vi "定点周期设置.vi"(10 "配置信息":T9, 11 "测试状态输入":T1) -> (2 "周期设置输出":T10, 3 "测试状态输出":T1)   [LabVIEW 2016, in "TimingControl.lvclass"]
uses:
  TimingControl.lvclass
  <vilib>/Utility/miscctls.llb/LVPointTypeDef.ctl
panel:
  in  "每月启动":T3
  in  "每周启动":T2
  out "测试状态.结束时间":timestamp caption="结束时间" format="%<%y/%m/%d %H:%M:%S>T"
  out "测试状态.启动次数":dbl caption="启动次数"
  out "测试状态.启动时间":timestamp caption="启动时间" format="%<%y/%m/%d %H:%M:%S>T"
  in  "测量参数":T5 items=["氨氮"]
  out "保存输出":bool
  in  "保存":bool
  in  "退出":bool
  in  "批量设置":bool
  out "周期模式选择卡":enum32{"选项卡 1", "选项卡 2"}(tab)
  in  "定点周期":T6
  in  "间隔启动":T8
  in  "周期模式":T4
  # "分钟"
  # "次"
  # "分钟"
  # "次"
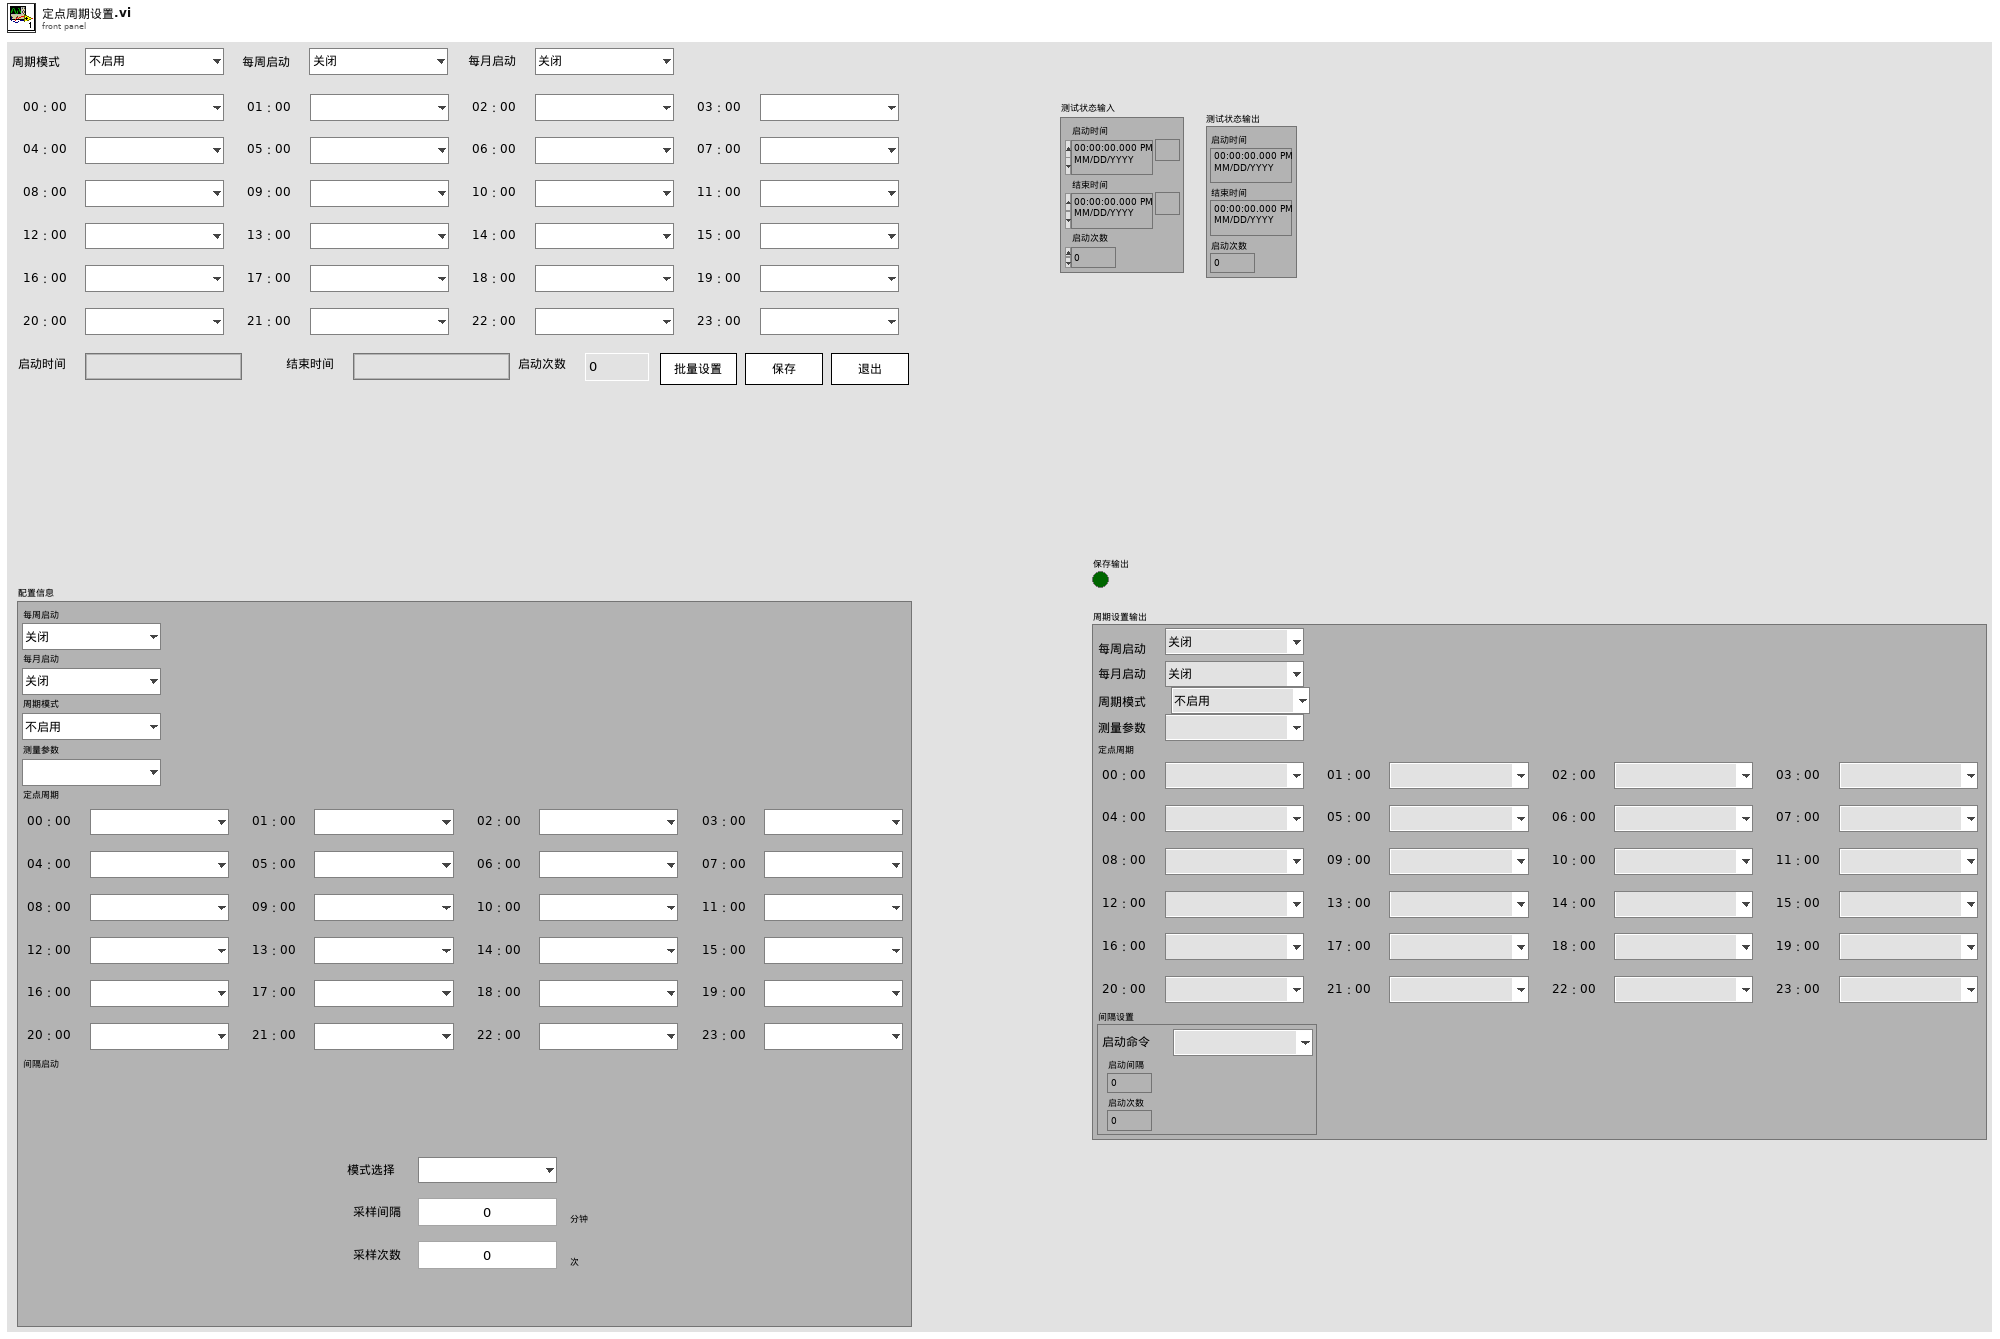
[diagram p1: front panel]
types:
  T1 = cluster{"启动时间":timestamp, "结束时间":timestamp, "启动次数":dbl}
  T2 = typedef "TimingControl.lvclass/每周启动.ctl" = enum16{"关闭", "周日", "周一", "周二", "周三", "周四", "周五", "周六"}
  T3 = typedef "TimingControl.lvclass/每月启动.ctl" = enum16{"关闭", "1号", "2号", "3号", "4号", "5号", "6号", "7号", "8号", "9号", "10号", "11号", "12号", "13号", "14号", "15号", "16号", "17号", "18号", "19号", "20号", "21号", "22号", "23号", "24号", "25号", "26号", "27号", "28号", "29号", "30号", "31号"}
  T4 = typedef "TimingControl.lvclass/周期模式设置.ctl" = enum16{"不启用", "定点模式", "间隔模式"}
  T5 = typedef "TimingControl.lvclass/测量参数.ctl" = u16
  T6 = typedef "TimingControl.lvclass/定点周期设置.ctl" = cluster{"启动命令":T7, "启动命令 2":T7, "启动命令 3":T7, "启动命令 4":T7, "启动命令 5":T7, "启动命令 6":T7, "启动命令 7":T7, "启动命令 8":T7, "启动命令 9":T7, "启动命令 10":T7, "启动命令 11":T7, "启动命令 12":T7, "启动命令 13":T7, "启动命令 14":T7, "启动命令 15":T7, "启动命令 16":T7, "启动命令 17":T7, "启动命令 18":T7, "启动命令 19":T7, "启动命令 20":T7, "启动命令 21":T7, "启动命令 22":T7, "启动命令 23":T7, "启动命令 24":T7}
  T7 = typedef "TimingControl.lvclass/启动命令选择.ctl" = enum16{"", "水样测试", "标样核查", "零点核查", "跨度核查", "空白测试", "平行样测试", "加标回收", "空白校准", "标样校准", "初始化(清洗)"}
  T8 = typedef "TimingControl.lvclass/间隔启动设置.ctl" = cluster{"启动命令":T7, "启动间隔":dbl, "启动次数":i32}
  T9 = cluster{"每周启动":T2, "每月启动":T3, "周期模式":T4, "测量参数":T5, "定点周期":T6, "间隔启动":T8}
  T10 = cluster{"每周启动":T2, "每月启动":T3, "周期模式":T4, "测量参数":T5, "定点周期":T6, "间隔设置":cluster{"启动命令":T7, "启动间隔":dbl, "启动次数":i32}}
  T11 = typedef "LVPointTypeDef.ctl" = cluster{"Horizontal":i16, "Vertical":i16}
  T12 = typedef "周期设置.lvlib/周期模式设置.ctl" = enum16{"不启用", "定点模式", "间隔模式"}
  T13 = cluster{"每周启动":T2, "每月启动":T3, "周期模式":T4, "测量参数":T5, "定点周期":T6, cluster{"启动命令":T7, "启动间隔":dbl, "启动次数":i32}}
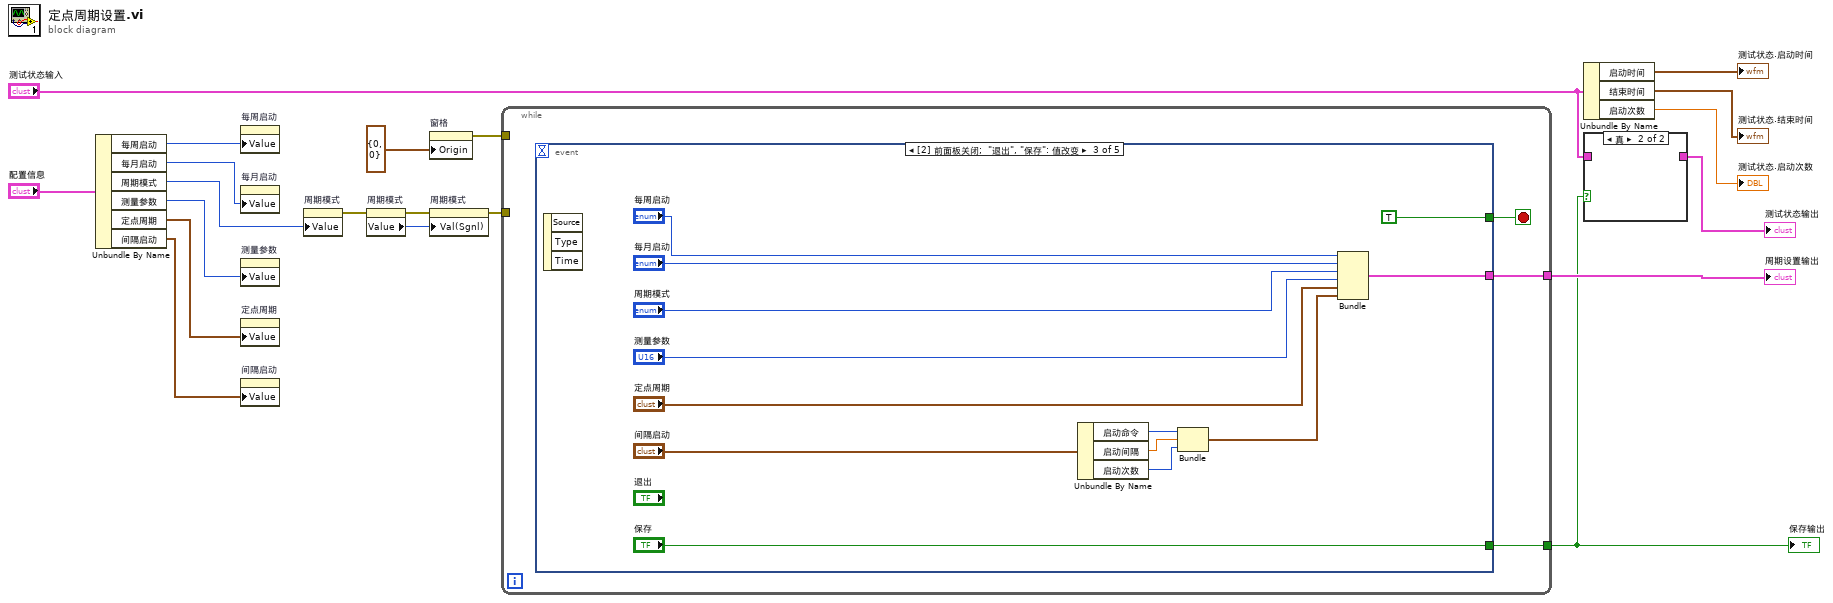
[diagram p0: block diagram]
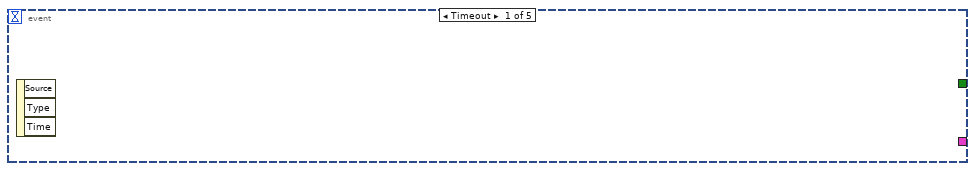
[diagram p3: hidden frame]
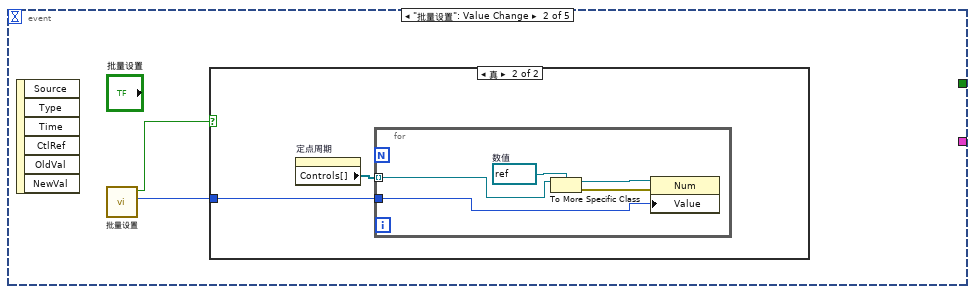
[diagram p4: hidden frame]
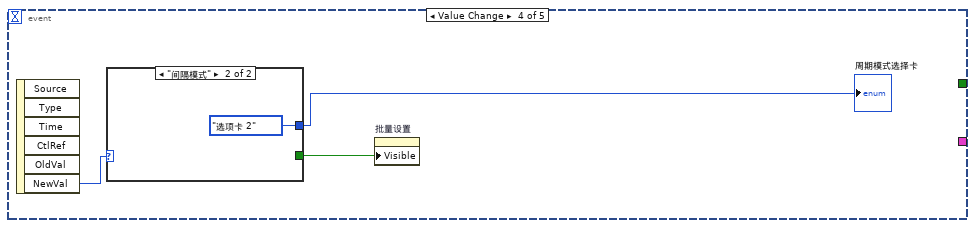
[diagram p6: hidden frame]
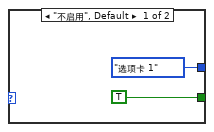
[diagram p7: hidden frame]
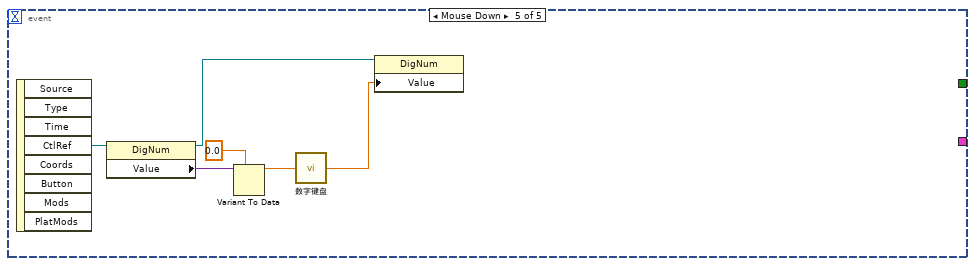
[diagram p8: hidden frame]
diagram:
  n1 = Unbundle By Name("配置信息") -> ("每周启动"=w9:T2, "每月启动"=w8:T3, "周期模式"=w10:T4, "测量参数"=w7:T5, "定点周期"=w6:T6, "间隔启动"=w5:T8)
  n2 = property on="每周启动" class="Enum (严格)"("Value"=w9) -> ()  [unwired: 2 in, 2 out]
  n3 = property on="每月启动" class="Enum (严格)"("Value"=w8) -> ()  [unwired: 2 in, 2 out]
  n4 = property on="测量参数" class="Ring (严格)"("Value"=w7) -> ()  [unwired: 2 in, 2 out]
  n5 = property on="定点周期" class="Clust (严格)"("Value"=w6) -> ()  [unwired: 2 in, 2 out]
  n6 = property on="间隔启动" class="Clust (严格)"("Value"=w5) -> ()  [unwired: 2 in, 2 out]
  n7 = property on="周期模式" class="Enum (严格)"("Value"=w10) -> (error out=w4:errorcluster)  [unwired: 2 in, 1 out]
  n8 = property on="周期模式" class="Enum (严格)"(error in=w4) -> (error out=w19:errorcluster, "Value"=w20:T12)  [unwired: 1 in, 1 out]
  n9 = property on="窗格" class="Pane"("Origin"=T11 {"Horizontal"=0, "Vertical"=0} ("原点")) -> (error out=w12:errorcluster)  [unwired: 2 in, 1 out]
  n10 = property on="周期模式" class="Enum (严格)"(error in=w19, "Val(Sgnl)"=w20) -> (error out=w18:errorcluster)  [unwired: 1 in, 1 out]
  n11 = while {
    tunnel: [w22] -> w17
    tunnel: w18 -> [_]
    tunnel: [w21] -> w2
    tunnel: w12 -> [_]
    stop <- w23 stop-if-true
    n12 = event shown="[2] 前面板关闭;  \"退出\", \"保存\": 值改变" {
      selector: _ -> [_ _ _ _ _]
      dyn-events: _ -> [_ _ _ _ _]
      timeout: _ -> [_ _ _ _ _]
      tunnel: [_ _ TRUE _ _] -> w23
      tunnel: [_ _ w44 _ _] -> w22
      tunnel: [_ _ "保存" _ _] -> w21
      event Timeout {
        n13 = event-data() -> ()  [unwired: 1 in, 3 out]
      }
      event "批量设置": Value Change {
        n14 = event-data() -> ()  [unwired: 1 in, 6 out]
        n15 = call "批量设置.vi"() -> ("启动命令 2"=w25:T7, "确定 2"=w24:bool)  [unwired: 10 in]
        n16 = case shown="真" w24 {
          tunnel: w25 -> [_ w26]
          frame False {
          }
          frame True {
            n17 = property on="定点周期" class="Clust (严格)"() -> ("Controls[]"=w27:refnum<vi>[])  [unwired: 2 in, 2 out]
            n18 = for {
              tunnel: w27 -> [w32] mode=indexing
              tunnel: w26 -> [w28]
              w31 = refnum<vi> refnum  # 数值
              n19 = To More Specific Class(target class=w31, reference=w32) -> (specific class reference=w30:refnum<vi>, error out=w29:errorcluster)  [unwired: 1 in]
              n20 = property class="Num"(reference=w30, error in=w29, "Value"=w28) -> ()  [unwired: 2 out]
            }
          }
        }
      }
      event Panel Close; "退出", "保存": Value Change {
        n21 = event-data() -> ()  [unwired: 1 in, 3 out]
        n22 = Unbundle By Name("间隔启动") -> ("启动命令"=w41:T7, "启动间隔"=w40:dbl, "启动次数"=w39:i32)
        n23 = Bundle("启动命令"=w41, "启动间隔"=w40, "启动次数"=w39) -> (w38:cluster{"启动命令":T7, "启动间隔":dbl, "启动次数":i32})  [unwired: 1 in]
        n24 = Bundle("每周启动"="每周启动", "每月启动"="每月启动", "周期模式"="周期模式", "测量参数"="测量参数", "定点周期"="定点周期", w38) -> (w44:T13)  [unwired: 1 in]
      }
      event Value Change {
        n25 = event-data() -> ("NewVal"=w47:T4)  [unwired: 1 in, 5 out]
        n26 = case shown="\"间隔模式\"" w47 {
          tunnel: [TRUE ("可见") _] -> w48
          tunnel: [enum32{"选项卡 1", "选项卡 2"}."选项卡 1" ("周期模式选择卡") enum32{"选项卡 1", "选项卡 2"}."选项卡 2" ("周期模式选择卡")] -> w46
          frame "不启用", Default {
          }
          frame "间隔模式" {
          }
        }
        "周期模式选择卡" <- w46
        n27 = property on="批量设置" class="Bool"("Visible"=w48) -> ()  [unwired: 2 in, 2 out]
      }
      event Mouse Down {
        n28 = event-data() -> ("CtlRef"=w57:refnum<vi>)  [unwired: 1 in, 7 out]
        n29 = property class="DigNum"(reference=w57) -> (reference out=w56:refnum<vi>, "Value"=w55:variant)  [unwired: 1 in, 1 out]
        n30 = Variant To Data(type=0.0, Variant=w55) -> (data=w53:dbl)  [unwired: 1 in, 1 out]
        n31 = call "数字键盘.vi"("OldNumber"=w53) -> ("NewNumber"=w52:sgl)
        n32 = property class="DigNum"(reference=w56, "Value"=w52) -> ()  [unwired: 1 in, 2 out]
      }
    }
  }
  "周期设置输出" <- w17
  "保存输出" <- w2
  n33 = Unbundle By Name("测试状态输入") -> ("启动时间"=→"测试状态.启动时间":timestamp, "结束时间"=→"测试状态.结束时间":timestamp, "启动次数"=→"测试状态.启动次数":dbl)
  n34 = case shown="真" w2 {
    tunnel: "测试状态输入" -> [w58 _]
    tunnel: [w58 _] -> w1
    frame False {
    }
    frame True {
    }
  }
  "测试状态输出" <- w1
